vi "Destroy to Session.vi"(8 "Error In":errorcluster, 10 "File Info":refnum<class "File Info.lvclass">, 11 "Session In":refnum<class "Session.lvclass">) -> (0 "Error Out":errorcluster, 3 "Session Out":refnum<class "Session.lvclass">)   [LabVIEW 2021, in "Field_RnD_Services_LIBSSH2_Toolkit.lvlib" / "File Info.lvclass"]
doc: "Passes through the Session object and destroys this File Info object."
uses:
  220524-VNA RP FLAT.llb/File Info.lvclass
  220524-VNA RP FLAT.llb/Session.lvclass
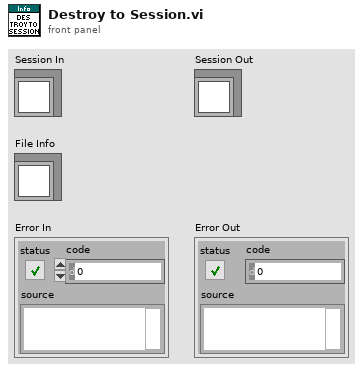
[diagram p1: front panel]
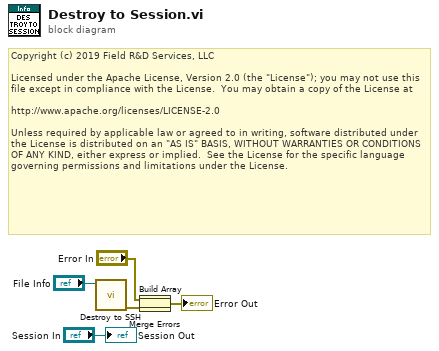
[diagram p0: block diagram]
diagram:
  # "Copyright (c) 2019 Field R&D Services, LLC\n\nLicensed under the Apache License, Version 2.0 (the \"License\"); you may not use this file except in compliance with the License.  You may obtain a copy of the License at\n\nhttp://www.apache.org/licenses/LICENSE-2.0\n\nUnless required by applicable law or agreed to in writing, software distributed under the License is distributed on an \"AS IS\" BASIS, WITHOUT WARRANTIES OR CONDITIONS OF ANY KIND, either express or implied.  See the License for the specific language governing permissions and limitations under the License."
  n1 = call "Destroy to SSH.vi"("File Info"="File Info") -> ("Error Out"=w2:errorcluster)  [unwired: 9 in, 1 out]
  n2 = Build Array("Error In", w2) -> (w1:errorcluster[])
  n3 = Merge Errors(w1) -> (→"Error Out":errorcluster)
  "Session Out" <- "Session In"
